vi "exercice7-2.vi"() -> ()   [LabVIEW 2013]
panel:
  out "error":string
  out "reponse":string
  in  "message":string
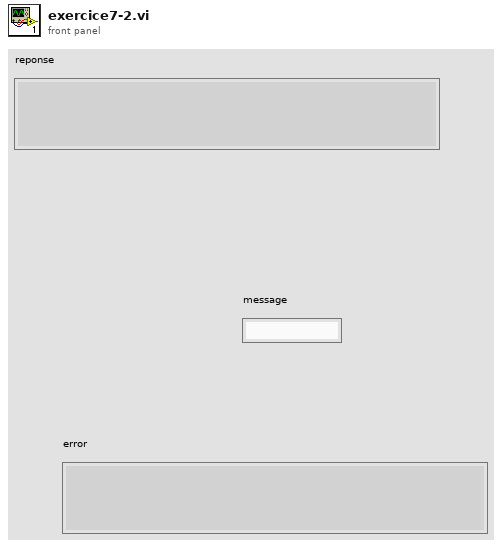
[diagram p1: front panel]
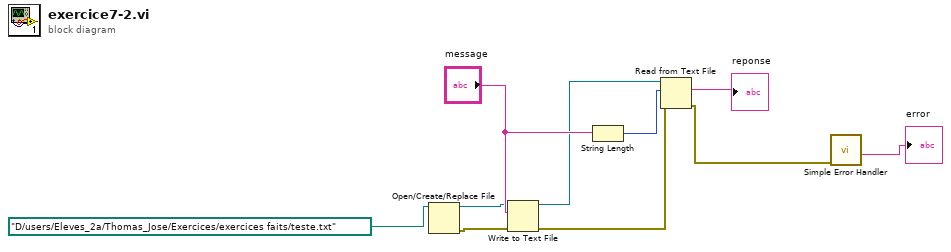
[diagram p0: block diagram]
diagram:
  n1 = Open/Create/Replace File(file path (use dialog)=path "D:/users/Eleves_2a/Thomas_Jose/Exercices/exercices faits/teste.txt") -> (refnum out=w5:refnum<file>, error out=w2:errorcluster)  [unwired: 5 in, 1 out]
  n2 = Write to Text File(file (use dialog)=w5, text="message", error in=w2) -> (refnum out=w4:refnum<file>, error out=w3:errorcluster)  [unwired: 1 in, 1 out]
  n3 = String Length(string="message") -> (length=w7:i32)
  n4 = Read from Text File(file (use dialog)=w4, count=w7, error in=w3) -> (text=→"reponse":string, error out=w6:errorcluster)  [unwired: 1 in, 2 out]
  n5 = call <vilib>:"Simple Error Handler.vi"("error in (no error)"=w6) -> ("source out"=→"error":string)  [unwired: 4 in, 4 out]
